vi "Config protocol settings from meas config.vi"(11 "measurement configuration":T2={"Weighting filter"="Linear", "Full scale range"=2.825, "Channel name"="", "Analog source resource name"="", "Frequency"=0.0, "Amplitude"=0.0, "Protocol capture resource name"="", "Data line"=0, "Interferer channel"=0, "Victim channel"=0, "Sample rate"=44100.0, "Measurement duration"=0.1, "Frame sync edge for channel 0"=1, "Channel count per frame"=2, "Channel length"=32, "Bit depth"=24, "Channel 0 offset"=1, "Endianness"=0, "Data justification"=0, "Frame length"=64, "Frame sync pulse width"=32, "Bit clock edge sync"=1}) -> (3 "Protocol settings":T1={"Protocol capture resource name"="", "Data line"=0, "Channel"="", "Clock rate"=12288000, "Number of words"=19200, "Sensitivity"=0.34762, "Frame sync edge for channel 0"=enum."Falling", "Channel count per frame"=2, "Channel length"=32, "Bit depth"=24, "Channel 0 offset"=1, "Endianness"=enum."MSB First", "Data justification"=enum."Left Justified", "Frame length"=64, "Frame sync pulse width"=32, "Bit clock edge sync"=enum."Falling"})   [LabVIEW 2021, in "crosstalk_Audio ADC.lvlib"]
uses:
  crosstalk_Audio ADC.lvlib
  Measurement Configuration.ctl
  shared/controls/Protocol Settings Dual Channel.ctl
  shared/controls/Audio ADC Controls.lvlib
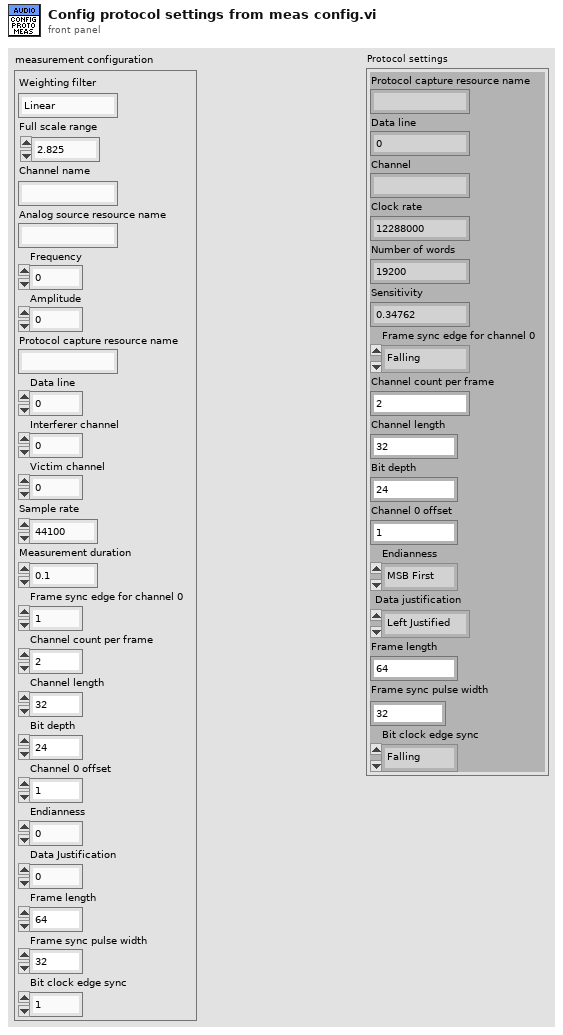
[diagram p1: front panel]
types:
  T1 = typedef "Audio ADC Controls.lvlib/Protocol Settings Dual Channel.ctl" = cluster{"Protocol capture resource name":string, "Data line":u16, "Channel":string, "Clock rate":u32, "Number of words":i32, "Sensitivity":dbl, "Frame sync edge for channel 0":enum32{"Rising", "Falling"}, "Channel count per frame":u8, "Channel length":u16, "Bit depth":u8, "Channel 0 offset":u16, "Endianness":enum32{"MSB First", "LSB First"}, "Data justification":enum32{"Left Justified", "Right Justified"}, "Frame length":u16, "Frame sync pulse width":u16, "Bit clock edge sync":enum32{"Rising", "Falling"}}
  T2 = typedef "Crosstalk_Audio ADC.lvlib/Measurement Configuration.ctl" = cluster{"Weighting filter":string, "Full scale range":dbl, "Channel name":string, "Analog source resource name":string, "Frequency":dbl, "Amplitude":dbl, "Protocol capture resource name":string, "Data line":u32, "Interferer channel":u32, "Victim channel":u32, "Sample rate":dbl, "Measurement duration":dbl, "Frame sync edge for channel 0":u32, "Channel count per frame":u32, "Channel length":u32, "Bit depth":u32, "Channel 0 offset":u32, "Endianness":u32, "Data justification":u32, "Frame length":u32, "Frame sync pulse width":u32, "Bit clock edge sync":u32}
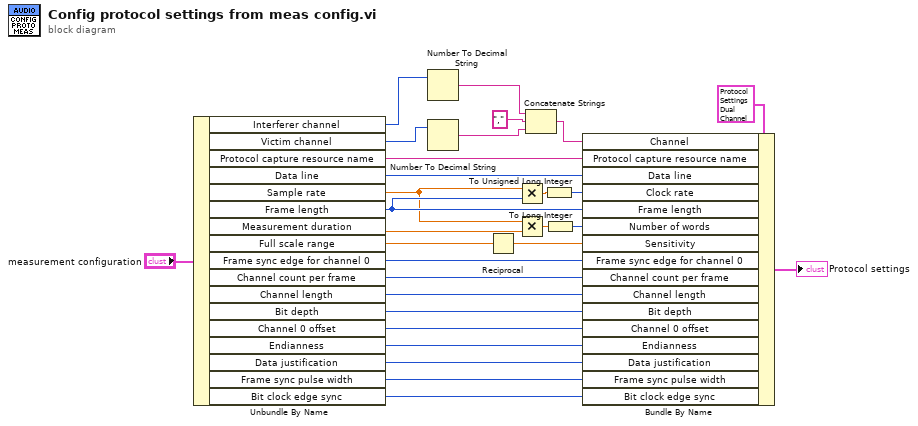
[diagram p0: block diagram]
diagram:
  n1 = Unbundle By Name("measurement configuration") -> ("Interferer channel"=w6:u32, "Victim channel"=w5:u32, "Protocol capture resource name"=w28:string, "Data line"=w27:u32, "Sample rate"=w13:dbl, "Frame length"=w15:u32, "Measurement duration"=w14:dbl, "Full scale range"=w10:dbl, "Frame sync edge for channel 0"=w18:u32, "Channel count per frame"=w26:u32, "Channel length"=w25:u32, "Bit depth"=w24:u32, "Channel 0 offset"=w23:u32, "Endianness"=w22:u32, "Data justification"=w21:u32, "Frame sync pulse width"=w20:u32, "Bit clock edge sync"=w19:u32)
  n2 = Number To Decimal String(number=w6) -> (decimal integer string=w3:string)  [unwired: 1 in]
  n3 = Number To Decimal String(number=w5) -> (decimal integer string=w1:string)  [unwired: 1 in]
  n4 = Reciprocal(x=w10) -> (1/x=w9:dbl)
  n5 = Multiply(x=w13, y=w15) -> (x*y=w17:dbl)
  n6 = Multiply(x=w13, y=w14) -> (x*y=w12:dbl)
  n7 = Concatenate Strings(w3, "," ("string"), w1) -> (w4:string)
  n8 = To Unsigned Long Integer(number=w17) -> (unsigned 32bit integer=w16:u32)
  n9 = To Long Integer(number=w12) -> (32bit integer=w11:i32)
  n10 = Bundle By Name(cluster=T1 {"Protocol capture resource name"="", "Data line"=0, "Channel"="", "Clock rate"=12288000, "Number of words"=19200, "Sensitivity"=0.34762, "Frame sync edge for channel 0"=enum."Falling", "Channel count per frame"=2, "Channel length"=32, "Bit depth"=24, "Channel 0 offset"=1, "Endianness"=enum."MSB First", "Data justification"=enum."Left Justified", "Frame length"=64, "Frame sync pulse width"=32, "Bit clock edge sync"=enum."Falling"} ("Protocol settings"), "Channel"=w4, "Protocol capture resource name"=w28, "Data line"=w27, "Clock rate"=w16, "Frame length"=w15, "Number of words"=w11, "Sensitivity"=w9, "Frame sync edge for channel 0"=w18, "Channel count per frame"=w26, "Channel length"=w25, "Bit depth"=w24, "Channel 0 offset"=w23, "Endianness"=w22, "Data justification"=w21, "Frame sync pulse width"=w20, "Bit clock edge sync"=w19) -> (→"Protocol settings":T1)
